vi "Query with no type.vi"(8 "error in (no error)":errorcluster, 9 "Type":variant, 10 "Query string":string, 11 "mysql in":refnum<class "mysql.lvclass">) -> (0 "error out":errorcluster, 2 "Variant":variant, 3 "mysql out":refnum<class "mysql.lvclass">)   [LabVIEW 2020, in "mysql.lvlib" / "mysql.lvclass"]
uses:
  mysql.lvclass
  7ccc19a8-9064-4274-ab4c-fae0e080c18f.vi
  private/Mysql command.vi
  private/Mysql data reader Scalar string.vi
  private/ping connection and reopen if needed.vi
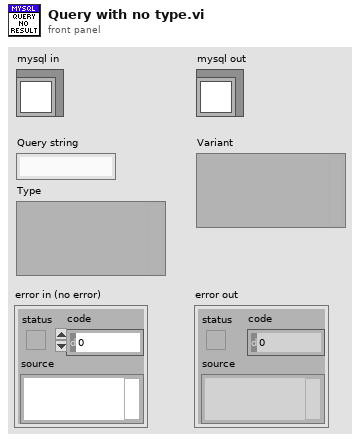
[diagram p1: front panel]
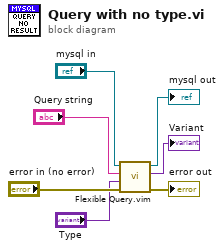
[diagram p0: block diagram]
diagram:
  n1 = call "Flexible Query.vim"("error in (no error)"="error in (no error)", "Type in"="Type", "Query string"="Query string", "mysql in"="mysql in") -> ("error out"=→"error out":errorcluster, "Result"=→"Variant":variant, "mysql out"=→"mysql out":refnum<class "mysql.lvclass">)  [unwired: 5 in]
